vi "Write Permeation Tube.vi"(8 "error in (no error)":errorcluster, 10 "Permeation Tube":T1 {"Molecular Weight" min=0.0 format="%#_3g"; "Permeation Rate \n(ng/min)" min=0; "Calibration Temperature\n(Celcius)" min=0}, 11 "Owlstone GEN-SYS in":refnum<class "Owlstone GEN-SYS.lvclass">) -> (0 "error out":errorcluster, 3 "Owlstone GEN-SYS out":refnum<class "Owlstone GEN-SYS.lvclass">)   [LabVIEW 2011, in "Owlstone GEN-SYS.lvclass"]
uses:
  Owlstone GEN-SYS.lvclass
  Permeation Tube.ctl
  Permeation Tube Gas.ctl
  Owlstone GEN-SYS.lvclass/Owlstone GEN-SYS.ctl
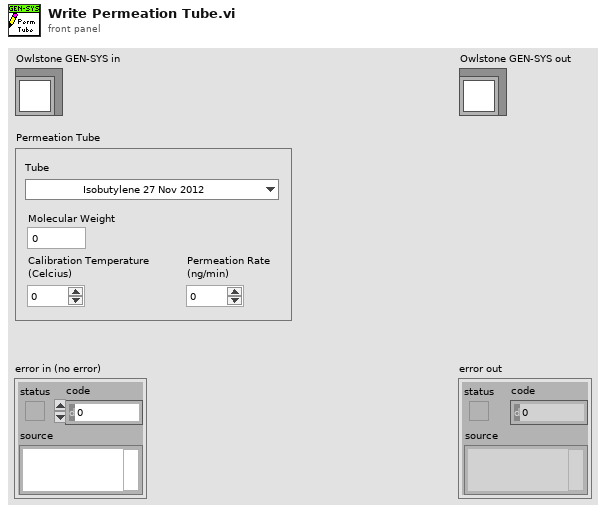
[diagram p1: front panel]
types:
  T1 = typedef "Owlstone GEN-SYS.lvclass/Permeation Tube.ctl" = cluster{"Tube":T2, "Molecular Weight":dbl, "Calibration Temperature\n(Celcius)":i32, "Permeation Rate \n(ng/min)":i32}
  T2 = typedef "Owlstone GEN-SYS.lvclass/Permeation Tube Gas.ctl" = enum16{"Isobutylene 27 Nov 2012", "Ammonia 29 Sep 2012", "DMMP Tube A 3 July 2014", "DMMP Tube B 3 July 2014"}
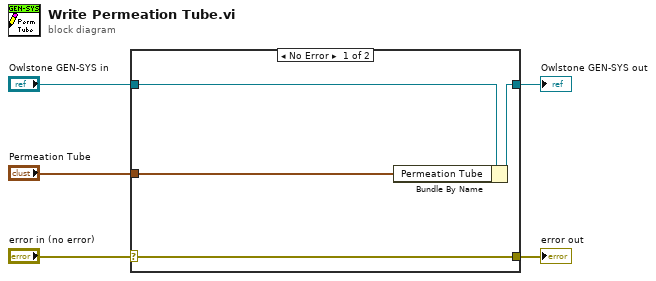
[diagram p0: block diagram]
diagram:
  n1 = case shown="No Error" "error in (no error)" {
    selector: "error in (no error)" -> [w9 w10]
    tunnel: [w9 w10] -> w4
    tunnel: [w7 w11] -> w2
    tunnel: "Owlstone GEN-SYS in" -> [w8 w11]
    tunnel: "Permeation Tube" -> [w6 _]
    frame No Error {
      n2 = Bundle By Name(cluster=w8, "Permeation Tube"=w6) -> (w7:refnum<class "Owlstone GEN-SYS.lvclass">)
    }
    frame Error {
    }
  }
  "error out" <- w4
  "Owlstone GEN-SYS out" <- w2
